vi "Fix path [polymorphic].vi"   [LabVIEW 2015, in "RT Management.lvlib" / "File Transfer Behavior.lvclass"]
uses:
  File Transfer Behavior.lvclass
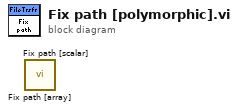
[diagram p0: block diagram]
diagram:
  n1 = call "Fix path [array].vi"() -> ()  [unwired: 9 in, 3 out]
  n2 = call "Fix path [scalar].vi"() -> ()  [unwired: 9 in, 3 out]
